vi "BC Major Frame Instructions.vi"(8 "error in (no error)":errorcluster, 11 "Bus Controller in":refnum<class "Bus Controller.lvclass">) -> (0 "error out":errorcluster, 3 "Bus Controller out":refnum<class "Bus Controller.lvclass">)   [LabVIEW 2020, in "Unit Tests.lvlib" / "Bus Controller.lvclass"]
uses:
  Bus Controller.lvclass
  Data Pointers.ctl
  Bus Controller.lvclass/Bus Controller.ctl
  Dependencies/Registry/Registry.lvclass/Registry.ctl
  Frames & Messages/TypeDefs/BC Op Codes - Verbose.ctl
  Frames & Messages/TypeDefs/BC Condition Codes.ctl
  <vilib>/addons/_JKI Toolkits/Caraya/classes/Assert/Assert True.vi
  Dependencies/FPGA Interface/FPGA Interface.lvclass
  BCI-1553 API.lvlib
  <vilib>/addons/_JKI Toolkits/Caraya/classes/Assert/Assert.lvclass
  Dependencies/Registry/Registry.lvclass
  <vilib>/addons/_JKI Toolkits/Caraya/classes/Test/Test.lvclass
panel:
  out "Array":T1[](array[typedef])
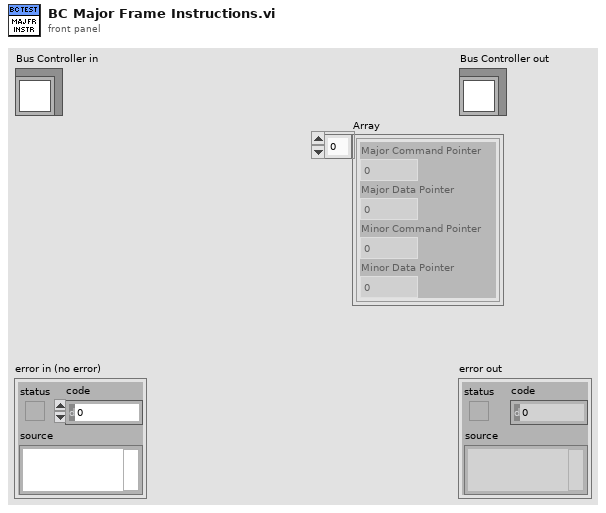
[diagram p1: front panel]
types:
  T1 = typedef "Data Pointers.ctl" = cluster{"Major Command Pointer":u16, "Major Data Pointer":u16, "Minor Command Pointer":u16, "Minor Data Pointer":u16}
  T2 = typedef "BCI-1553 API.lvlib/BC Condition Codes.ctl" = enum16{"GP0 == 1 || LT", "GP1 == 1 || NE", "GP2 == 1", "GP3 == 1", "GP4 == 1", "GP5 == 1", "GP6 == 1", "GP7 == 1", "NORESP", "FMTERR", "GOODBLOCK", "MSKSTATSET", "BADMSG", "1RETRY", "2RETRY", "ALWAYS"}
  T3 = typedef "BCI-1553 API.lvlib/BC Op Codes - Verbose.ctl" = enum16{"EXECUTE MSG", "EXECUTE MSG GO", "JUMP", "CALL SUBROUTINE", "RETURN", "INTERRUPT REQUEST", "HALT", "DELAY", "WAIT FRAME TIMER = 0", "COMPARE FRAME TIMER", "COMPARE MSG TIMER", "LOAD TIME TAG CTR", "LOAD TIME TAG CTR HI", "LOAD FRAME TIMER", "START FRAME TIMER", "PUSH TIME TAG COUNT", "PUSH TIME TAG COUNT HI", "PUSH TIME TAG COUNT BOTH", "PUSH BLOCK STATUS WORD", "PUSH CURRENT VALUE", "PUSH INDIRECT", "WAIT EXT TRIGGER", "EXECUTE AND FLIP", "EXECUTE, FLIP, GO", "WRITE VALUE TO WMI", "WRITE VALUE TO MEM", "DECREMENT RAM, SKIP", "FLAG"}
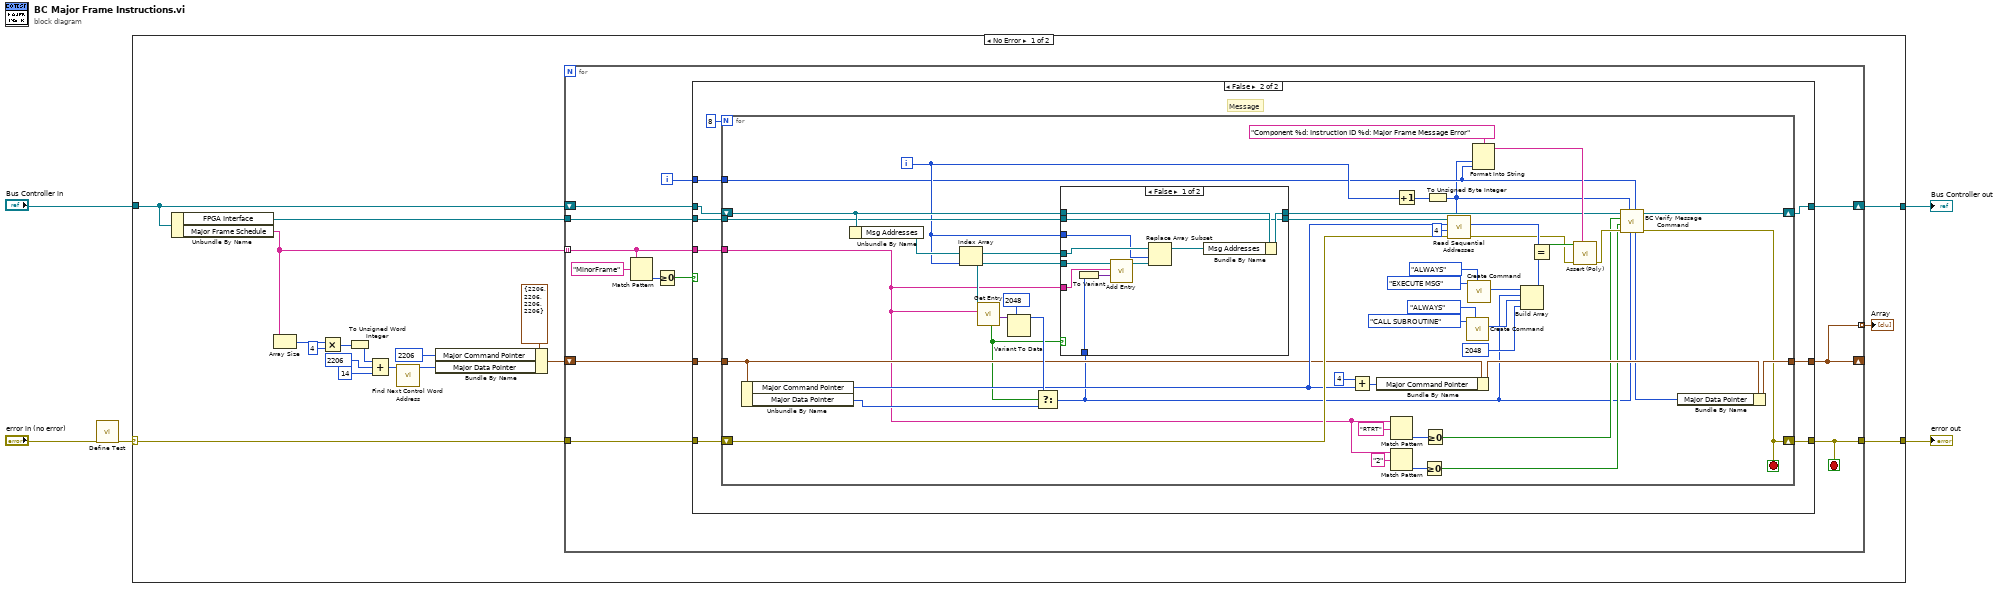
[diagram p0: block diagram]
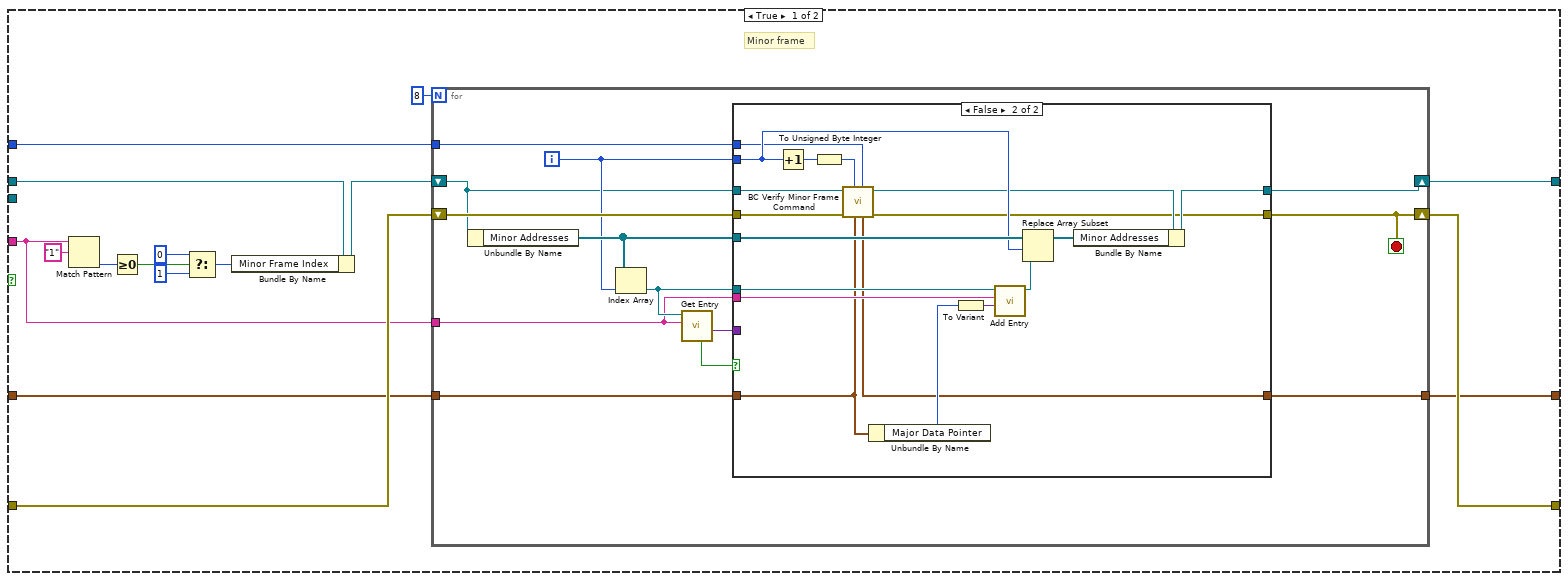
[diagram p2: hidden frame]
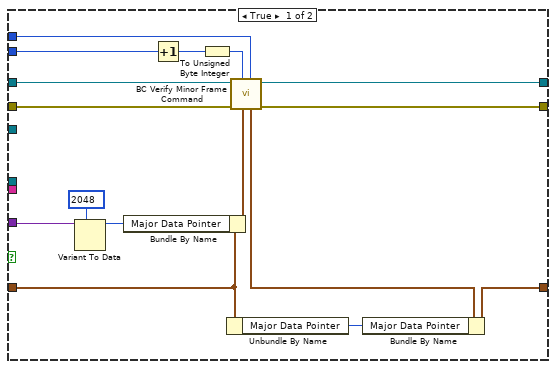
[diagram p3: hidden frame]
diagram:
  n1 = call <vilib>:"Define Test.vi"("error in (no error)"="error in (no error)") -> ("error out"=w2:errorcluster)  [unwired: 9 in, 1 out]
  n2 = case shown="No Error" w2 {
    selector: w2 -> [w11 w171]
    tunnel: [w10 w171] -> w5
    tunnel: [w8 w170] -> w3
    tunnel: "Bus Controller in" -> [w9 w170]
    frame No Error {
      n3 = Unbundle By Name(w9) -> ("FPGA Interface"=w13:refnum<class "FPGA Interface.lvclass">, "Major Frame Schedule"=w12:string[])
      n4 = Array Size(array=w12) -> (size(s)=w22:i32)
      n5 = Multiply(x=w22, y=4) -> (x*y=w20:i32)
      n6 = To Unsigned Word Integer(number=w20) -> (unsigned 16bit integer=w19:u16)
      n7 = Compound Arithmetic op=ADD(w19, u16 2206, u16 14 ("y")) -> (w17:u16)
      n8 = call "Find Next Control Word Address.vi"("Starting Address"=w17) -> ("0xHHHX Address"=w15:u16)  [unwired: 10 in]
      n9 = Bundle By Name(cluster=T1 {"Major Command Pointer"=2206, "Major Data Pointer"=2206, "Minor Command Pointer"=2206, "Minor Data Pointer"=2206}, "Major Command Pointer"=u16 2206, "Major Data Pointer"=w15) -> (w14:T1)
      n10 = for {
        tunnel: w11 -> [w35]
        tunnel: [w33] -> w10
        tunnel: w13 -> [w34]
        tunnel: w12 -> [w29] mode=indexing
        shift-right: [w24] -> _
        shift-left: w14 -> [w27]
        shift-right: [w25] -> w8
        shift-left: w9 -> [w26]
        tunnel: [w24] -> w7 mode=indexing
        i -> [w28]
        stop <- w33 stop-if-true
        n11 = Match Pattern(string=w29, regular expression="MinorFrame") -> (offset past match=w31:i32)  [unwired: 1 in, 3 out]
        n12 = Greater Or Equal To 0?(x=w31) -> (x >= 0?=w30:bool)
        n13 = case shown="False" w30 {
          tunnel: [w36 w108] -> w25
          tunnel: w35 -> [w50 w106]
          tunnel: [w49 w105] -> w33
          tunnel: w34 -> [_ w104]
          tunnel: w29 -> [w39 w103]
          tunnel: w28 -> [w51 w107]
          tunnel: w27 -> [w41 w101]
          tunnel: [w40 w100] -> w24
          tunnel: w26 -> [w38 w99]
          frame True {
            # "Minor frame"
            n14 = Match Pattern(string=w39, regular expression="1") -> (offset past match=w47:i32)  [unwired: 1 in, 3 out]
            n15 = Greater Or Equal To 0?(x=w47) -> (x >= 0?=w46:bool)
            n16 = Select(t=0 ("Minor Frame Index"), s=w46, f=1 ("Minor Frame Index")) -> (s? t:f=w44:i32)
            n17 = Bundle By Name(cluster=w38, "Minor Frame Index"=w44) -> (w37:refnum<class "Bus Controller.lvclass">)
            n18 = for {
              N: 8 -> [_]
              tunnel: w51 -> [w62]
              shift-right: [w64] -> w49
              shift-left: w50 -> [w60]
              tunnel: w41 -> [w61]
              tunnel: [w63] -> w40
              tunnel: w39 -> [w55]
              shift-right: [w52] -> w36
              shift-left: w37 -> [w57]
              i -> [w58]
              stop <- w64 stop-if-true
              n19 = Unbundle By Name(w57) -> ("Minor Addresses"=w59:refnum<class "Registry.lvclass">[])
              n20 = Index Array(array=w59, index=w58) -> (element=w56:refnum<class "Registry.lvclass">)
              n21 = call "Get Entry.vi"("Key"=w55, "Registry in"=w56) -> ("Value"=w53:variant, "Found?"=w54:bool)  [unwired: 6 in, 2 out]
              n22 = case shown="False" w54 {
                tunnel: [w71 w94] -> w52
                tunnel: [w65 w85] -> w64
                tunnel: [w74 w84] -> w63
                tunnel: w62 -> [w70 w82]
                tunnel: w61 -> [w75 w83]
                tunnel: w57 -> [w72 w88]
                tunnel: w60 -> [w66 w86]
                tunnel: w53 -> [w78 _]
                tunnel: w56 -> [_ w92]
                tunnel: w58 -> [w77 w96]
                tunnel: w59 -> [_ w97]
                tunnel: w55 -> [_ w91]
                frame True {
                  n23 = Variant To Data(type=u16 2048, Variant=w78) -> (data=w76:u16)  [unwired: 1 in, 1 out]
                  n24 = Bundle By Name(cluster=w75, "Major Data Pointer"=w76) -> (w67:T1)
                  n25 = Increment(x=w77) -> (x+1=w80:i32)
                  n26 = To Unsigned Byte Integer(number=w80) -> (unsigned 8bit integer=w69:u8)
                  n27 = Unbundle By Name(w75) -> ("Major Data Pointer"=w73:u16)
                  n28 = call "BC Verify Minor Frame Command.vi"("Instruction ID"=w70, "Pointers"=w67, "Target IC (1-8)"=w69, "error in (no error)"=w66, "Bus Controller in"=w72) -> ("error out"=w65:errorcluster, "Bus Controller out"=w71:refnum<class "Bus Controller.lvclass">, "Pointers out"=w68:T1)  [unwired: 4 in]
                  n29 = Bundle By Name(cluster=w68, "Major Data Pointer"=w73) -> (w74:T1)
                }
                frame False {
                  n30 = Increment(x=w96) -> (x+1=w98:i32)
                  n31 = To Unsigned Byte Integer(number=w98) -> (unsigned 8bit integer=w81:u8)
                  n32 = call "BC Verify Minor Frame Command.vi"("Instruction ID"=w82, "Pointers"=w83, "Target IC (1-8)"=w81, "error in (no error)"=w86, "Bus Controller in"=w88) -> ("error out"=w85:errorcluster, "Bus Controller out"=w87:refnum<class "Bus Controller.lvclass">, "Pointers out"=w84:T1)  [unwired: 4 in]
                  n33 = Unbundle By Name(w83) -> ("Major Data Pointer"=w93:u16)
                  n34 = To Variant(anything=w93) -> (Variant=w90:variant)
                  n35 = call "Add Entry.vi"("Value"=w90, "Key"=w91, "Registry in"=w92) -> ("Registry out"=w89:refnum<class "Registry.lvclass">)  [unwired: 6 in, 2 out]
                  n36 = Replace Array Subset(array=w97, new element=w89, index=w96) -> (w95:refnum<class "Registry.lvclass">[])
                  n37 = Bundle By Name(cluster=w87, "Minor Addresses"=w95) -> (w94:refnum<class "Bus Controller.lvclass">)
                }
              }
            }
          }
          frame False {
            # "Message"
            n38 = for {
              N: 8 -> [_]
              tunnel: w107 -> [w119]
              tunnel: w104 -> [w147]
              tunnel: w103 -> [w112]
              shift-right: [w120] -> w105
              shift-left: w106 -> [w156]
              shift-right: [w122] -> w108
              shift-left: w99 -> [w148]
              tunnel: w101 -> [w129]
              tunnel: [w127] -> w100
              i -> [w133]
              stop <- w120 stop-if-true
              n39 = Unbundle By Name(w129) -> ("Major Command Pointer"=w131:u16, "Major Data Pointer"=w132:u16)
              n40 = Unbundle By Name(w148) -> ("Msg Addresses"=w134:refnum<class "Registry.lvclass">[])
              n41 = Index Array(array=w134, index=w133) -> (element=w113:refnum<class "Registry.lvclass">)
              n42 = call "Get Entry.vi"("Key"=w112, "Registry in"=w113) -> ("Value"=w111:variant, "Found?"=w110:bool)  [unwired: 6 in, 2 out]
              n43 = Variant To Data(type=u16 2048, Variant=w111) -> (data=w149:u16)  [unwired: 1 in, 1 out]
              n44 = Select(t=w149, s=w110, f=w132) -> (s? t:f=w114:u16)
              n45 = case shown="False" w110 {
                tunnel: w134 -> [w163 _]
                tunnel: w112 -> [w158 _]
                tunnel: w114 -> [w167 _]
                tunnel: [w164 w169] -> w146
                tunnel: w147 -> [w164 w169]
                tunnel: [w165 w168] -> w123
                tunnel: w148 -> [w166 w168]
                tunnel: w113 -> [w160 _]
                tunnel: w133 -> [w161 _]
                frame False {
                  n46 = To Variant(anything=w167) -> (Variant=w157:variant)
                  n47 = call "Add Entry.vi"("Value"=w157, "Key"=w158, "Registry in"=w160) -> ("Registry out"=w159:refnum<class "Registry.lvclass">)  [unwired: 6 in, 2 out]
                  n48 = Replace Array Subset(array=w163, new element=w159, index=w161) -> (w162:refnum<class "Registry.lvclass">[])
                  n49 = Bundle By Name(cluster=w166, "Msg Addresses"=w162) -> (w165:refnum<class "Bus Controller.lvclass">)
                }
                frame True {
                }
              }
              n50 = Add(x=u16 4 ("y"), y=w131) -> (x+y=w130:u16)
              n51 = Bundle By Name(cluster=w129, "Major Command Pointer"=w130) -> (w128:T1)
              n52 = Match Pattern(string=w112, regular expression="RTRT") -> (offset past match=w151:i32)  [unwired: 1 in, 3 out]
              n53 = Match Pattern(string=w112, regular expression="2") -> (offset past match=w154:i32)  [unwired: 1 in, 3 out]
              n54 = Increment(x=w133) -> (x+1=w135:i32)
              n55 = Greater Or Equal To 0?(x=w154) -> (x >= 0?=w116:bool)
              n56 = Greater Or Equal To 0?(x=w151) -> (x >= 0?=w117:bool)
              n57 = To Unsigned Byte Integer(number=w135) -> (unsigned 8bit integer=w118:u8)
              n58 = call-dynamic "Read Sequential Addresses.vi"("Target IC (1-8)"=w118, "error in (no error)"=w156, "Addresses to Read"=u16 4, "Starting Address"=w131, "FPGA Interface in"=w146) -> ("error out"=w125:errorcluster, "Data"=w137:u16[])  [unwired: 5 in]
              n59 = call "Create Command.vi"("Condition"=BC_Condition_Codes."ALWAYS", "Op Code"=BC_Op_Codes_-_Verbose."CALL SUBROUTINE") -> ("Instruction"=w140:u16)  [unwired: 8 in, 1 out]
              n60 = call "Create Command.vi"("Condition"=BC_Condition_Codes."ALWAYS", "Op Code"=BC_Op_Codes_-_Verbose."EXECUTE MSG") -> ("Instruction"=w139:u16)  [unwired: 8 in, 1 out]
              n61 = Format Into String(format string="Component %d: Instruction ID %d: Major Frame Message Error" ("message (\"\")"), w118, w119) -> (resulting string=w124:string)  [unwired: 2 in, 1 out]
              n62 = Build Array(w139, w114, w140, u16 2048) -> (w138:u16[])
              n63 = Equal?(x=w137, y=w138) -> (x = y?=w126:bool)
              n64 = call-poly <vilib>:"Assert (Poly).vi"("Label"=w124, "error in (no error)"=w125, "True?"=w126) -> ("error out"=w121:errorcluster)  [unwired: 7 in, 1 out]
              n65 = call "BC Verify Message Command.vi"("Instruction ID"=w119, "Cmd Address"=w114, "Target IC (1-8)"=w118, "error in (no error)"=w121, "Transmit?"=w116, "RT-RT?"=w117, "Bus Controller in"=w123) -> ("error out"=w120:errorcluster, "Bus Controller out"=w122:refnum<class "Bus Controller.lvclass">, "Post-Data Address"=w115:u16)  [unwired: 2 in]
              n66 = Bundle By Name(cluster=w128, "Major Data Pointer"=w115) -> (w127:T1)
            }
          }
        }
      }
      "Array" <- w7
    }
    frame Error {
    }
  }
  "error out" <- w5
  "Bus Controller out" <- w3
